vi "translateMotorStatus.vi"(0 "ACESDEController in":refnum<class "ACESDEController.lvclass">, 2 "actual value":u32, 5 "error in (no error)":errorcluster) -> (14 "ACESDEController out":refnum<class "ACESDEController.lvclass">, 16 "motion_state":T1=enum."CONST", 17 "other_states":T1[](array[typedef]), 19 "error out":errorcluster)   [LabVIEW 2013, in "classes.lvlib" / "ACESDEController.lvclass"]
uses:
  ACESDEController.lvclass
  common/controls/motor_status.ctl
  libraries/common.lvlib
panel:
  out "other states":bool[](array[boolean])
  out "motion state":bool[](array[boolean])
  out "actual bits":bool[](array[boolean])
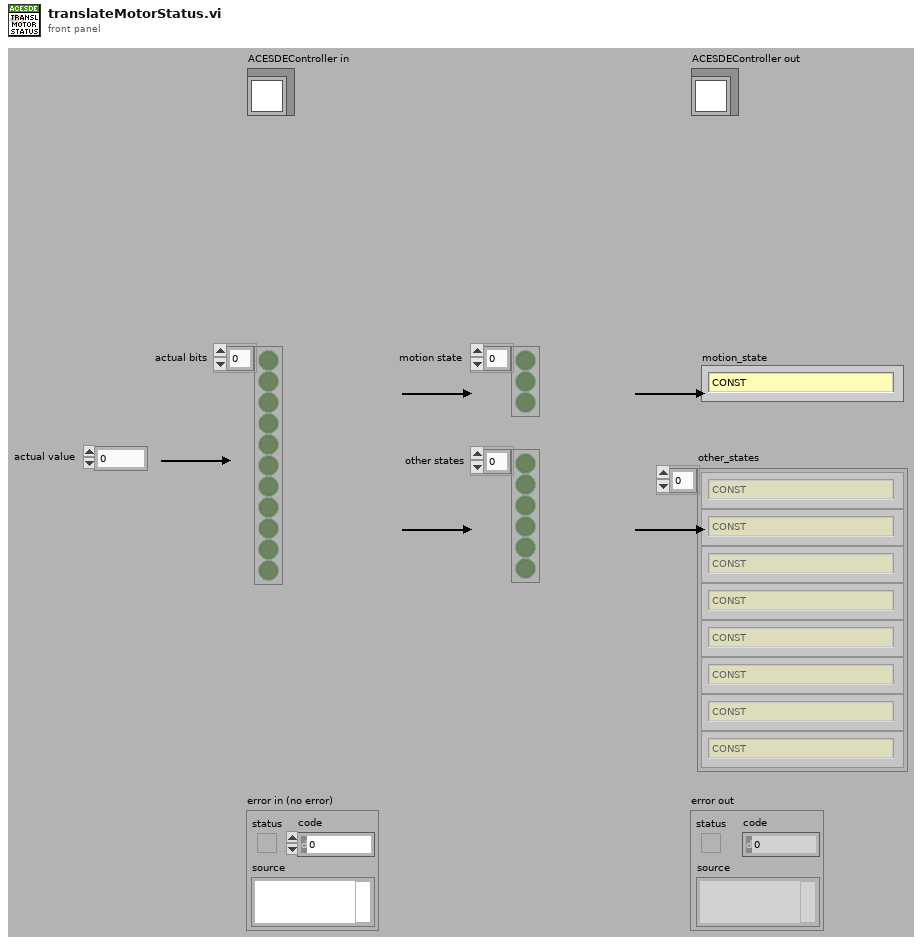
[diagram p1: front panel]
types:
  T1 = typedef "common.lvlib/motor_status.ctl" = enum16{"IDLE", "CONST", "ACCEL", "DECEL", "HOME_SWITCH", "-LIMIT_SWITCH", "+LIMIT_SWITCH", "-LIMIT_ERR", "+LIMIT_ERR", "COMM_TIMEOUT", "ALARM_INPUT", "ALARM_ERROR", "TOC_TIMEOUT_STATUS", "LATCH_INPUT_STATUS", "Z_INDEX_STATUS"}
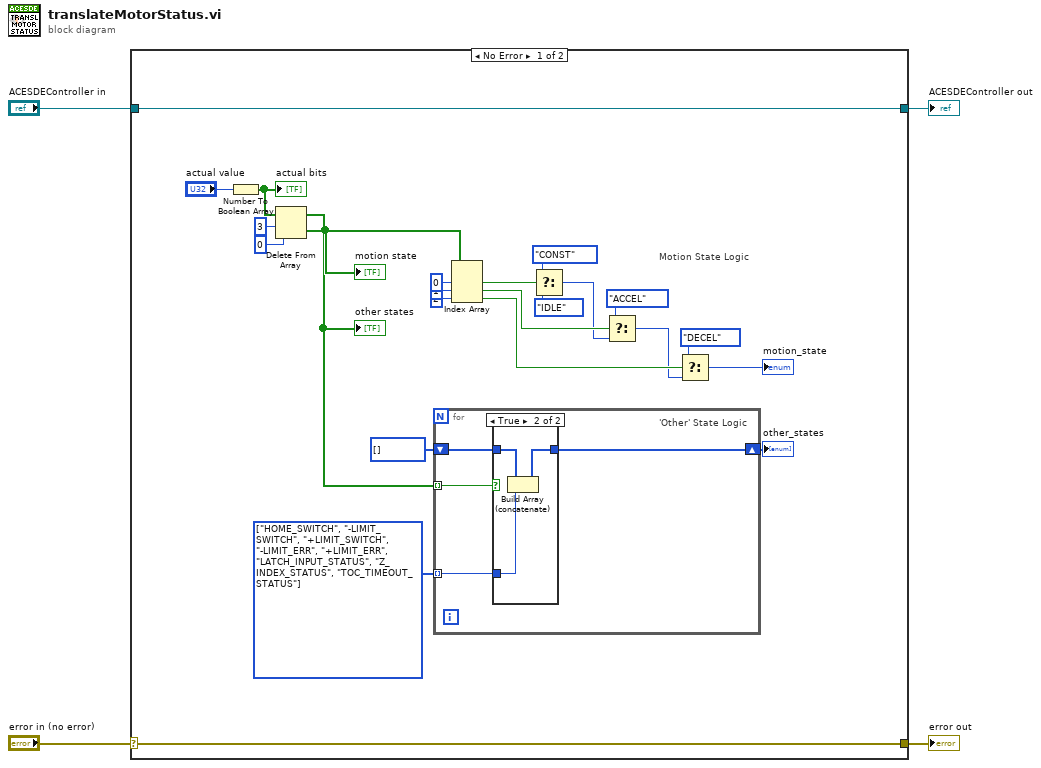
[diagram p0: block diagram]
diagram:
  n1 = case shown="No Error" "error in (no error)" {
    selector: "error in (no error)" -> [w27 w38]
    tunnel: [w27 w38] -> w3
    tunnel: [w28 w37] -> w1
    tunnel: "ACESDEController in" -> [w28 w37]
    frame No Error {
      w7 = T1[] [enum."HOME_SWITCH", enum."-LIMIT_SWITCH", enum."+LIMIT_SWITCH", enum."-LIMIT_ERR", enum."+LIMIT_ERR", enum."LATCH_INPUT_STATUS", enum."Z_INDEX_STATUS", enum."TOC_TIMEOUT_STATUS"] items=["IDLE", "CONST", "ACCEL", "DECEL", "HOME_SWITCH", "-LIMIT_SWITCH", "+LIMIT_SWITCH", "-LIMIT_ERR", "+LIMIT_ERR", "COMM_TIMEOUT", "ALARM_INPUT", "ALARM_ERROR", "TOC_TIMEOUT_STATUS", "LATCH_INPUT_STATUS", "Z_INDEX_STATUS"]
      w8 = T1[] [] items=["IDLE", "CONST", "ACCEL", "DECEL", "HOME_SWITCH", "-LIMIT_SWITCH", "+LIMIT_SWITCH", "-LIMIT_ERR", "+LIMIT_ERR", "COMM_TIMEOUT", "ALARM_INPUT", "ALARM_ERROR", "TOC_TIMEOUT_STATUS", "LATCH_INPUT_STATUS", "Z_INDEX_STATUS"]
      # "Motion State Logic"
      n2 = Number To Boolean Array(number="actual value") -> (Boolean array=w25:bool[])
      "actual bits" <- w25
      n3 = Delete From Array(array=w25, length=3, index=0) -> (deleted portion=w9:bool[], array with subset deleted=w5:bool[])
      "motion state" <- w9
      "other states" <- w5
      n4 = for {
        tunnel: w5 -> [w32] mode=indexing
        shift-right: [w29] -> w6
        shift-left: w8 -> [w31]
        tunnel: w7 -> [w30] mode=indexing
        # "'Other' State Logic"
        n5 = case shown="True" w32 {
          tunnel: w31 -> [w33 w36]
          tunnel: w30 -> [_ w35]
          tunnel: [w33 w34] -> w29
          frame False {
          }
          frame True {
            n6 = Build Array (concatenate)(w36, w35) -> (w34:T1[])
          }
        }
      }
      "other_states" <- w6
      n7 = Index Array(array=w9, index #1=0 ("index"), index #2=1 ("index"), index #3=2 ("index")) -> (element #1=w18:bool, element #2=w16:bool, element #3=w12:bool)
      n8 = Select(t=motor_status."CONST" ("motion_state"), s=w18, f=motor_status."IDLE" ("motion_state")) -> (s? t:f=w15:T1)
      n9 = Select(t=motor_status."ACCEL" ("motion_state"), s=w16, f=w15) -> (s? t:f=w11:T1)
      n10 = Select(t=motor_status."DECEL" ("motion_state"), s=w12, f=w11) -> (s? t:f=→"motion_state":T1)
    }
    frame Error {
    }
  }
  "error out" <- w3
  "ACESDEController out" <- w1
